vi "get Motion.vi"(11 "Ship in":refnum<class "Ship.lvclass">) -> (2 "Motion.lvclass":refnum<class "Motion.lvclass">, 3 "Ship out":refnum<class "Ship.lvclass">)   [LabVIEW 2015]
uses:
  Ship.lvclass
  Motion/Motion.lvclass
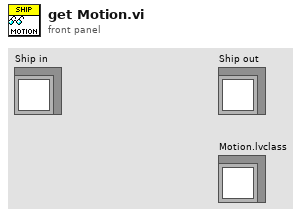
[diagram p1: front panel]
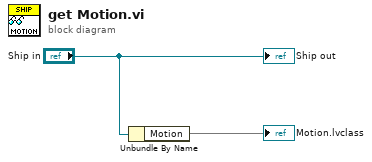
[diagram p0: block diagram]
diagram:
  n1 = Unbundle By Name("Ship in") -> ("Motion"=→"Motion.lvclass")
  "Ship out" <- "Ship in"
